vi "SPI_Transaction2.vi"(5 "Device":i32, 6 "Values to write":u8[](array[numeric]) format="%.0x", 7 "Bus":i32=1, 8 "error in":errorcluster, 10 "Delay (usec)":u32, 11 "Speed (Hz)":u32) -> (0 "error out":errorcluster, 4 "Values read":u8[](array[numeric]) format="%.0x")   [LabVIEW 2014]
doc: "Performs an SPI transaction (write/read) with the specified device. The chip select line is held between blocks."
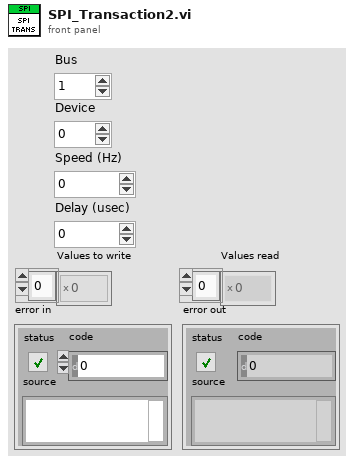
[diagram p1: front panel]
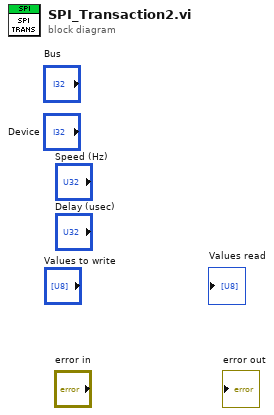
[diagram p0: block diagram]
diagram:
